vi "CSM - File Loader.vi"(5 "Init State(\"Macro: Initialize\")":string="Macro: Initialize", 7 "Name(\"\" to use uuid)":string="CSM Tiny") -> ()   [LabVIEW 2020]
doc: "Template for building CSM Module without User Interface.\n\n<b>Inputs:</b>\n- <b>Name(\"\" to use uuid)</b>: Module Name\n - If Input is \"\", an uuid will be used for module name. The module is marked as stand-alone mode and will not be included in module list.\n - Fi Input end with '#', the module will worked in worker mode. Modules with the same name will shared the same message queue. Any external message will be processed by one of the modules, depends on who is free.\n - Otherwise, the input string will be used as module name, which should be unique in system. CSM will go to \"Critical Error\" state if duplicated module name is used in system.\n\n<b>Outputs:</b>\n - N/A"
uses:
  <userlib>/_NEVSTOP/Communicable State Machine(CSM)/_Support/Priority Queue/Priority Queue.lvclass/Priority Queue.ctl
  a15cecde-ba48-478f-b3ee-ddca9c6ade3a.vi
  45794baa-ad44-4491-a68b-119a749fa817.vi
  8437d9df-e1d6-4259-972b-d18eb56eaa28.vi
  <userlib>/_NEVSTOP/Communicable State Machine(CSM)/_Support/Process/CSMP-Async Call.vi
  <userlib>/_NEVSTOP/Communicable State Machine(CSM)/_Support/GlobalEvent/GEvt-Generate Status Log.vi
  <userlib>/_NEVSTOP/Communicable State Machine(CSM)/_Support/Process/CSMP-Broadcast.vi
  <userlib>/_NEVSTOP/Communicable State Machine(CSM)/_Support/GlobalEvent/GEvt-Generate Interrupt Log.vi
  <userlib>/_NEVSTOP/Communicable State Machine(CSM)/_Support/GlobalEvent/GEvt-Generate Register Log.vi
  <userlib>/_NEVSTOP/Communicable State Machine(CSM)/_Support/Process/CSMP-Register Status.vi
  <userlib>/_NEVSTOP/Communicable State Machine(CSM)/_Support/GlobalEvent/GEvt-Generate Unregister Log.vi
  <userlib>/_NEVSTOP/Communicable State Machine(CSM)/_Support/Process/CSMP-Unregister Status.vi
  <userlib>/_NEVSTOP/Communicable State Machine(CSM)/_Support/Process/CSMP-Sync Call.vi
  <userlib>/_NEVSTOP/Communicable State Machine(CSM)/_Support/CSMQ/_CSMObj-Unlock.vi
  <userlib>/_NEVSTOP/Communicable State Machine(CSM)/_Support/Process/CSMP-PostPostMsg.vi
  <userlib>/_NEVSTOP/Communicable State Machine(CSM)/_Support/Process/CSMP-PostSendMsg.vi
  <userlib>/_NEVSTOP/Communicable State Machine(CSM)/_Support/CSMQ/_CSMObj-Lock State.vi
  <userlib>/_NEVSTOP/Communicable State Machine(CSM)/_Support/Common/Splite Reason String Part.vi
  <userlib>/_NEVSTOP/Communicable State Machine(CSM)/_Support/Common/Trim Single line Text.vi
  <userlib>/_NEVSTOP/Communicable State Machine(CSM)/_Support/CSMQ/_CSMOFGV Release.vi
  <userlib>/_NEVSTOP/Communicable State Machine(CSM)/_Support/Common/Remove Comments from Line.vi
  <userlib>/_NEVSTOP/Communicable State Machine(CSM)/_Support/Common/Splite Single-line Message.vi
  <userlib>/_NEVSTOP/Communicable State Machine(CSM)/_Support/Common/Parse Next Single-line State.vi
  <userlib>/_NEVSTOP/Communicable State Machine(CSM)/_Support/CSMQ/_CSMOFGV Dequeue.vi
  <userlib>/_NEVSTOP/Communicable State Machine(CSM)/_Support/CSMQ/_CSMObj-Log Error if in a Remote Session.vi
  <userlib>/_NEVSTOP/Communicable State Machine(CSM)/_Support/GlobalEvent/GEvt-Generate State Change Log.vi
  <userlib>/_NEVSTOP/Communicable State Machine(CSM)/_Support/GlobalEvent/GEvt-Generate Remaining States Log.vi
  <userlib>/_NEVSTOP/Communicable State Machine(CSM)/_Support/GlobalEvent/GEvt-Generate Module Destroyed Log.vi
  <userlib>/_NEVSTOP/Communicable State Machine(CSM)/_Support/GlobalEvent/GEvt-Generate Complete Log.vi
  <userlib>/_NEVSTOP/Communicable State Machine(CSM)/_Support/GlobalEvent/GEvt-Generate Module Created Log.vi
  <userlib>/_NEVSTOP/Communicable State Machine(CSM)/_Support/Common/Format Timestamp.vi
  <userlib>/_NEVSTOP/Communicable State Machine(CSM)/AdvanceAPI/CSM - Revert Arguments-Safe String.vi
  <userlib>/_NEVSTOP/Communicable State Machine(CSM)/AdvanceAPI/CSM - Make String Arguments Safe.vi
  <userlib>/_NEVSTOP/Communicable State Machine(CSM)/AdvanceAPI/CSM - Break Down Multiple States String.vi
  <userlib>/_NEVSTOP/Communicable State Machine(CSM)/AdvanceAPI/CSM - Compact Multiple States.vi
  <userlib>/_NEVSTOP/Communicable State Machine(CSM)/_Support/CSMQ/_CSMObj-Message Check.vi
  <userlib>/_NEVSTOP/Communicable State Machine(CSM)/_Support/CSMQ/_CSMObj-Enqueue Cross-Module Message.vi
  <userlib>/_NEVSTOP/Communicable State Machine(CSM)/_Support/CSMQ/_CSMOFGV Get.vi
  <userlib>/_NEVSTOP/Communicable State Machine(CSM)/_Support/FGV-BroadcastRegistry/Cache-Broadcast Registry Search Result.vi
  <userlib>/_NEVSTOP/Communicable State Machine(CSM)/AdvanceAPI/CSM - Register Status Change.vi
  <userlib>/_NEVSTOP/Communicable State Machine(CSM)/AdvanceAPI/CSM - Unregister Status Change.vi
  <userlib>/_NEVSTOP/Communicable State Machine(CSM)/_Support/Common/Hex Str to U8 Data.vi
  <userlib>/_NEVSTOP/Communicable State Machine(CSM)/_Support/Common/Concatenate State with Arguments.vi
  <userlib>/_NEVSTOP/Communicable State Machine(CSM)/_Support/Common/U8 Data to Hex Str.vi
  <userlib>/_NEVSTOP/Communicable State Machine(CSM)/_Support/Priority Queue/Dequeue Element.vi
  <userlib>/_NEVSTOP/Communicable State Machine(CSM)/AdvanceAPI/CSM - Keywords.vi
  <userlib>/_NEVSTOP/Communicable State Machine(CSM)/_Support/Priority Queue/Enqueue Element.vi
  <userlib>/_NEVSTOP/Communicable State Machine(CSM)/_Support/GlobalEvent/FGV-GlobalEventRef.vi
  <userlib>/_NEVSTOP/Communicable State Machine(CSM)/_Support/CSMQ/_CSMOFGV Obtain.vi
  <userlib>/_NEVSTOP/Communicable State Machine(CSM)/_Support/CSMQ/_CSMOFGV.vi
  <userlib>/_NEVSTOP/Communicable State Machine(CSM)/_Support/Error/CSM Not Allowed Message.vi
  <userlib>/_NEVSTOP/Communicable State Machine(CSM)/_Support/GlobalEvent/FGV-StatusChangeEventRef.vi
  <userlib>/_NEVSTOP/Communicable State Machine(CSM)/_Support/FGV-BroadcastRegistry/global-CSMQ FGV Change Flag.vi
  <userlib>/_NEVSTOP/Communicable State Machine(CSM)/_Support/FGV-BroadcastRegistry/global-Broadcast Cache Change Flag.vi
  <userlib>/_NEVSTOP/Communicable State Machine(CSM)/_Support/BroadcastRegistry/HelperVI/Broadcast Item Key.vi
  <userlib>/_NEVSTOP/Communicable State Machine(CSM)/_Support/FGV-BroadcastRegistry/FGV-BroadcastRegistry.vi
  <userlib>/_NEVSTOP/Communicable State Machine(CSM)/_Support/Message/Parse Register Message.vi
  <userlib>/_NEVSTOP/Communicable State Machine(CSM)/_Support/Message/Parse Unregister Message.vi
  <userlib>/_NEVSTOP/Communicable State Machine(CSM)/AdvanceAPI/CSM - Replace Substitution Marks in Messages.vi
  <userlib>/_NEVSTOP/Communicable State Machine(CSM)/addons/API-String-Arugments-Support/_Support/Convert API String Arguments to Data(variant).vi
  <userlib>/_NEVSTOP/Communicable State Machine(CSM)/addons/MassData-Parameter/_support/FGV-MassData.vi
  <userlib>/_NEVSTOP/Communicable State Machine(CSM)/Communicable State Machine.lvlib
  <userlib>/_NEVSTOP/Communicable State Machine(CSM)/addons/Loop-Support/CSM Loop Support.lvlib
panel:
  out "Snippets Count":i32
  out "text":string
  out "offset (in bytes)":i64 format="%.3p"
  out "size (in bytes)":i64 format="%.3p"
  out "State History":string
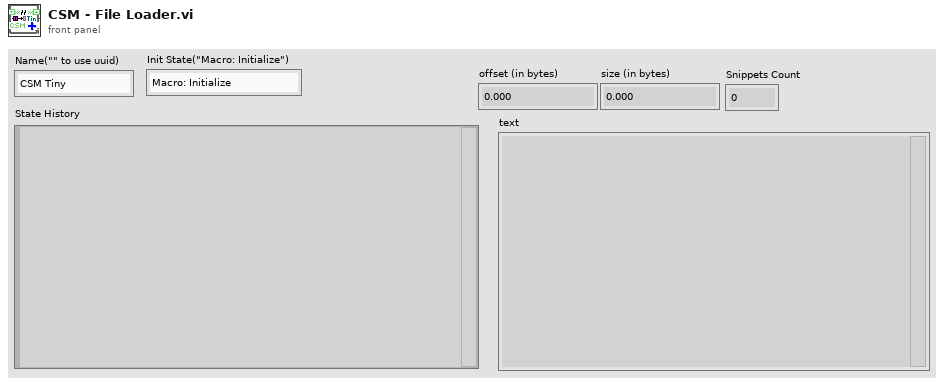
[diagram p1: front panel]
types:
  T1 = enum32{"Invalid", "Standard", "Closed", "Hidden", "Minimized", "Maximized"}
  T2 = enum32{"invalid app kind", "Development System", "Run Time System", "Student Edition", "Embedded LabVIEW", "Evaluation", "Custom"}
  T3 = typedef "Communicable State Machine.lvlib/_CSM_Response Source Message.ctl" = cluster{"‘State":string, "’Arguments":string, "’Error":errorcluster}
  T4 = cluster{"Core":cluster{"Current VI Reference":refnum<vi>, "Close Panel on Exit?":bool}, "Snippets Size":i32, "temp":string, "Snippets Count":i32}
  T5 = cluster{"Current VI Reference":refnum<vi>, "Close Panel on Exit?":bool}
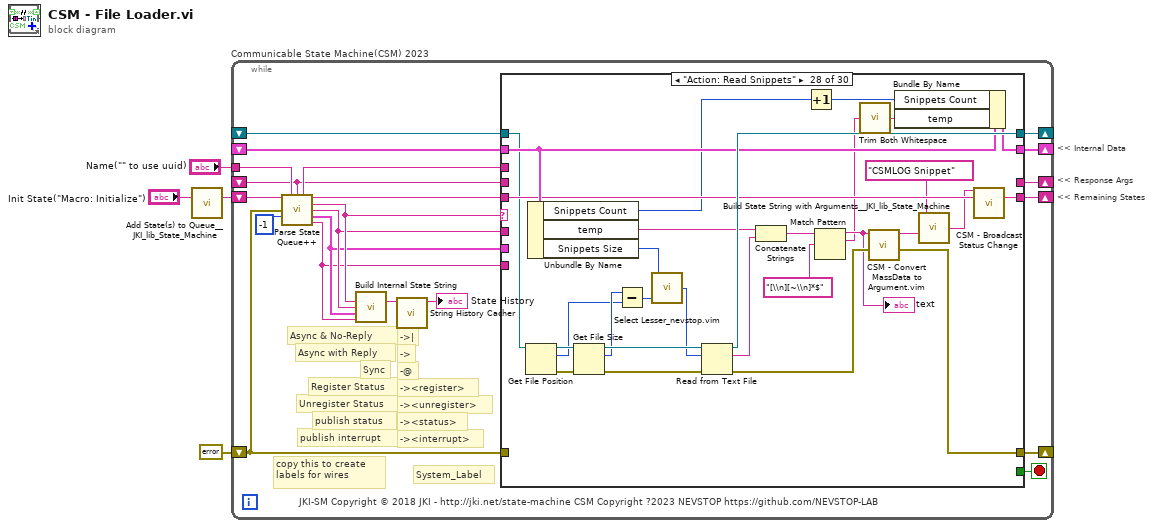
[diagram p0: block diagram]
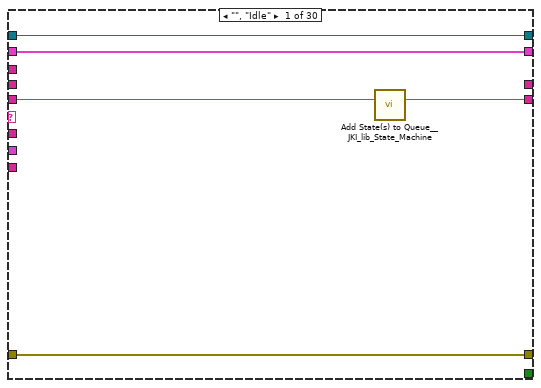
[diagram p2: hidden frame]
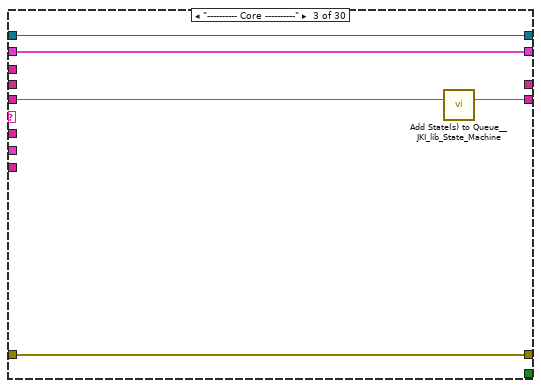
[diagram p4: hidden frame]
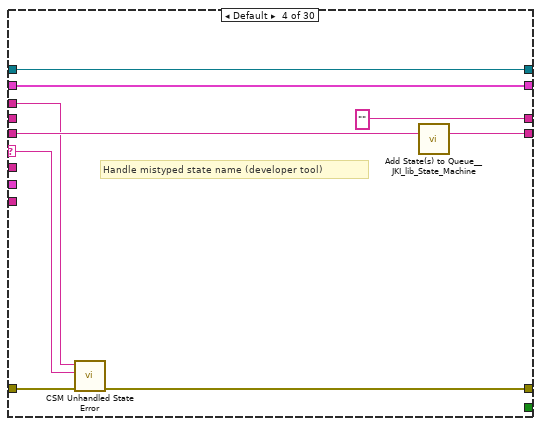
[diagram p5: hidden frame]
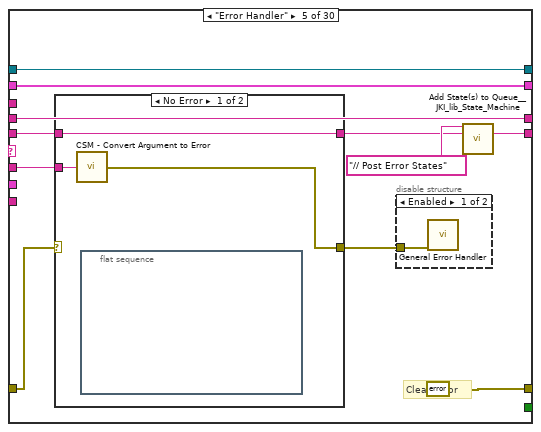
[diagram p6: hidden frame]
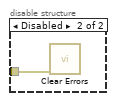
[diagram p7: hidden frame]
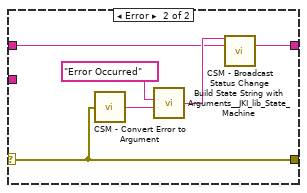
[diagram p8: hidden frame]
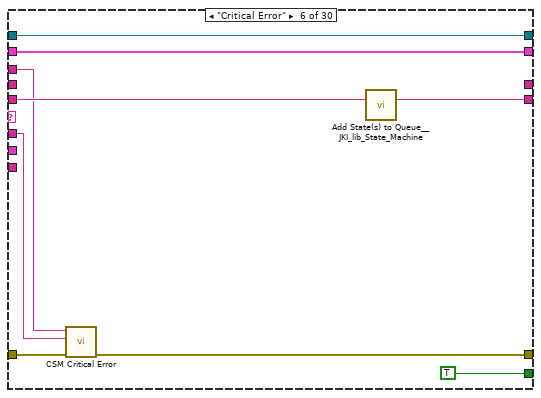
[diagram p9: hidden frame]
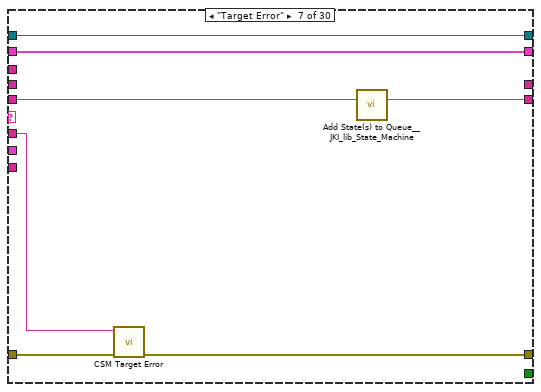
[diagram p10: hidden frame]
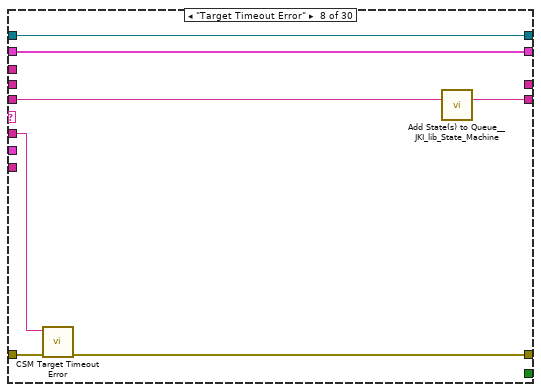
[diagram p11: hidden frame]
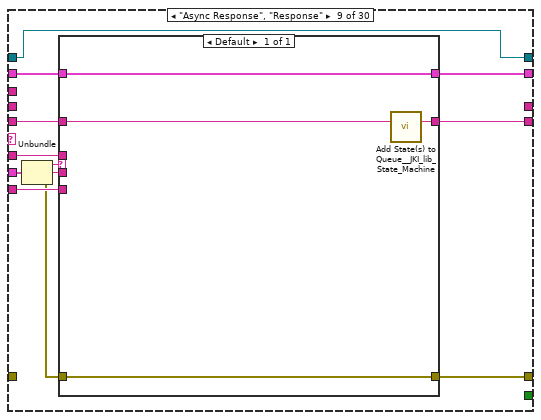
[diagram p12: hidden frame]
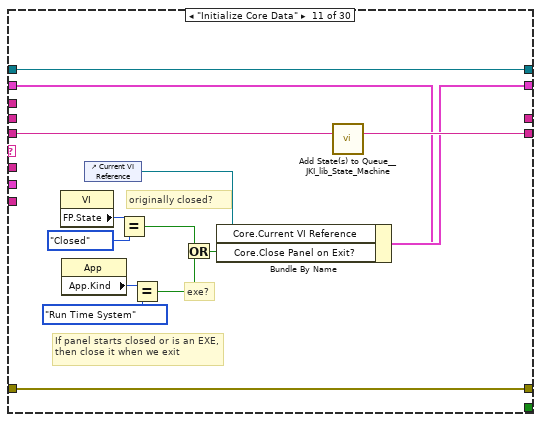
[diagram p14: hidden frame]
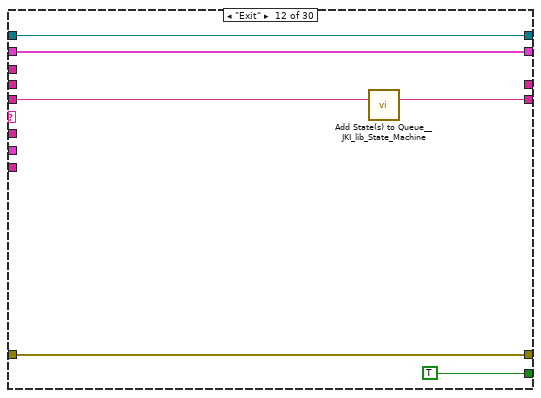
[diagram p15: hidden frame]
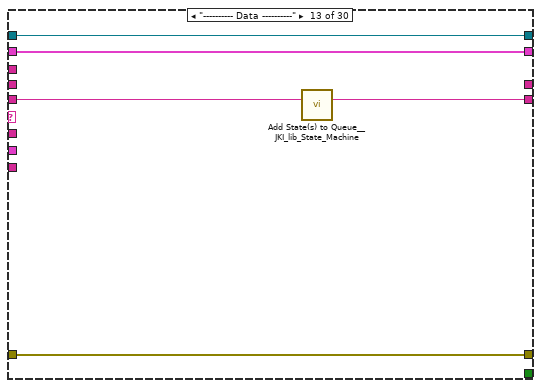
[diagram p16: hidden frame]
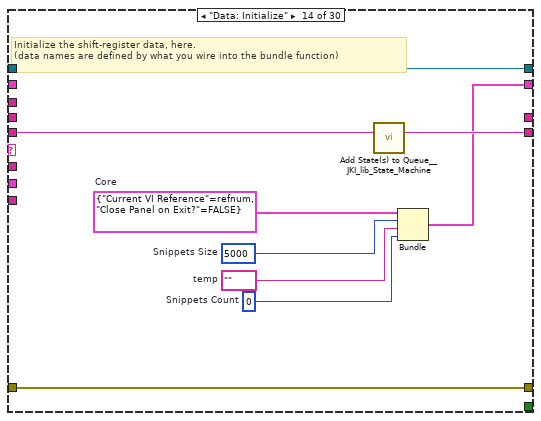
[diagram p17: hidden frame]
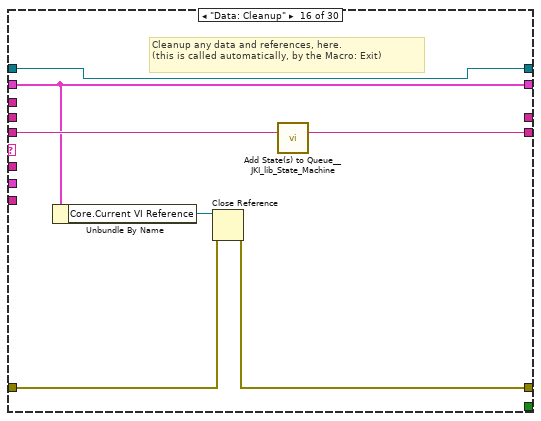
[diagram p19: hidden frame]
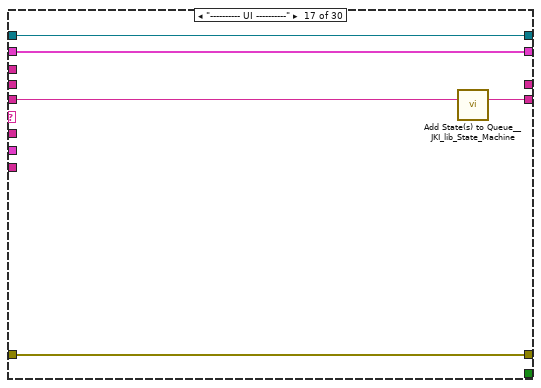
[diagram p20: hidden frame]
diagram:
  # "<< Internal Data"
  # "<< Response Args"
  # "<< Remaining States"
  n1 = call <vilib>:"Add State(s) to Queue__JKI_lib_State_Machine.vi"("State(s) in (\"\")"="Init State(\"Macro: Initialize\")") -> ("States Out"=w4:string)  [unwired: 14 in]
  n2 = while "Communicable State Machine(CSM) 2023" {
    shift-right: [w20] -> _
    shift-left: _ -> [w19]
    shift-right: [w23] -> _
    shift-left: errorcluster {"status"=FALSE, "code"=0, "source"=""} ("error out") -> [w18]
    shift-right: [w22] -> _
    shift-left: w4 -> [w24]
    tunnel: "Name(\"\" to use uuid)" -> [w16]
    shift-right: [w17] -> _
    shift-left: _ -> [w8]
    shift-right: [w6] -> _
    shift-left: _ -> [w5]
    stop <- w21 stop-if-true
    # "-><interrupt>"
    # "-><status>"
    # "-><unregister>"
    # "-><register>"
    # "-@"
    # "->"
    # "->|"
    # "publish interrupt"
    # "publish status"
    # "Unregister Status"
    # "Register Status"
    # "Sync"
    # "Async with Reply"
    # "Async & No-Reply"
    # "copy this to create labels for wires"
    # "System_Label"
    # "JKI-SM Copyright © 2018 JKI - http://jki.net/state-machine CSM Copyright ?2023 NEVSTOP https://github.com/NEVSTOP-LAB"
    n3 = call <userlib>:"Parse State Queue++.vi"("State Queue"=w24, "Name(\"\" to use uuid)"=w16, "Response Arguments"=w8, "Error In (no error)"=w18, "Dequeue Timeout(0ms)"=-1 ("Timeout")) -> ("Name Used"=w9:string, "Remaining States"=w25:string, "Current State"=w13:string, "Arguments"=w12:string, ">> Response Source Message >>"=w11:T3, ">> Source CSM >>"=w10:string)  [unwired: 5 in]
    n4 = call <userlib>:"Build Internal State String.vi"("State"=w13, "Arguments (\"\")"=w12, ">> Response Source Message >>"=w11, "Source (\"\")"=w10) -> ("State with Arguments"=w14:string)  [unwired: 11 in]
    n5 = call <userlib>:"String History Cacher.vi"("String"=w14) -> ("String Cache"=→"State History":string)  [unwired: 10 in]
    n6 = case shown="\"Action: Read Snippets\"" w13 {
      selector: w13 -> [_ _ _ w43 _ _ _ _ _ _ _ _ _ _ _ _ _ _ _ _ _ _ _ _ _ _ _ _ w346 _]
      tunnel: w25 -> [w27 w33 w39 w47 w55 w77 w84 w91 w100 w112 w127 w133 w138 w147 w150 w158 w163 w168 w175 w191 w261 w267 w275 w278 w288 w294 w305 w331 w348 w359]
      tunnel: w12 -> [_ _ _ _ w54 w73 w83 w89 w99 _ _ _ _ _ _ _ _ _ w170 w185 _ _ _ _ w282 _ w295 _ _ _]
      tunnel: w19 -> [w28 w32 w36 w45 w58 w78 w85 w92 w102 w111 w120 w131 w135 _ w149 w153 w160 w166 w173 w187 w258 w264 w272 w277 w287 w291 w303 w333 w336 w357]
      tunnel: [w29 w34 w37 w41 errorcluster {"status"=FALSE, "code"=0, "source"=""} ("error out") w74 w81 w88 w105 w113 w124 w130 w136 w144 w151 w154 w161 w165 w171 w188 w259 w265 w273 w279 w289 w292 w300 w329 w339 w355] -> w23
      tunnel: w18 -> [w29 w34 w37 w48 w56 w79 w82 w90 _ w113 w124 w130 w136 w144 w151 w155 w161 w165 w172 w189 w259 w265 w273 w279 w289 w292 _ _ _ _]
      tunnel: [w30 w33 w38 w46 w51 w76 w86 w93 w101 w112 w126 w132 w137 w146 w150 w157 w162 w167 w174 w190 w260 w266 w274 w278 w285 w293 w304 w332 w347 w358] -> w22
      tunnel: [_ _ _ _ _ TRUE _ _ _ _ _ TRUE _ _ _ _ _ _ _ _ _ _ _ _ _ _ _ _ _ _] -> w21
      tunnel: [w28 w32 w36 w45 w58 w78 w85 w92 w103 w111 w125 w131 w135 w145 w149 w153 w160 w166 w173 w187 w258 w264 w272 w277 w281 w291 w303 w314 w336 w357] -> w20
      tunnel: w10 -> [_ _ _ _ _ _ _ _ w97 _ _ _ _ _ _ _ _ _ _ _ _ _ _ _ _ _ _ _ _ _]
      tunnel: w11 -> [_ _ _ _ _ _ _ _ w104 _ _ _ _ _ _ _ _ _ _ _ _ _ _ _ _ _ _ _ _ _]
      tunnel: [_ _ _ "" w50 _ _ _ _ _ _ _ _ _ _ _ _ _ _ _ _ _ _ _ _ _ _ _ _ _] -> w17
      tunnel: w9 -> [_ _ _ w42 _ w72 _ _ _ _ _ _ _ _ _ _ _ _ _ _ _ _ _ _ _ _ _ _ _ _]
      tunnel: w8 -> [_ _ _ _ w50 _ _ _ _ _ _ _ _ _ _ _ _ _ _ _ _ _ _ _ _ _ _ _ _ _]
      tunnel: [w26 w31 w35 w40 w49 w71 w80 w87 w94 w110 w114 w128 w134 w141 w148 w152 w159 w164 w169 w184 w257 w262 w268 w276 w286 w290 w299 w334 w345 refnum<file> refnum ("refnum out")] -> w6
      tunnel: w5 -> [w26 w31 w35 w40 w49 w71 w80 w87 w94 w110 w114 w128 w134 w141 w148 w152 w159 w164 w169 w184 w257 w262 w268 w276 w286 w290 _ w326 w344 w356]
      frame "", "Idle" {
        n7 = call <vilib>:"Add State(s) to Queue__JKI_lib_State_Machine.vi"("State(s) in (\"\")"=w27) -> ("States Out"=w30:string)  [unwired: 14 in]
      }
      frame "CSM Documentation" {
      }
      frame "---------- Core ----------" {
        n8 = call <vilib>:"Add State(s) to Queue__JKI_lib_State_Machine.vi"("State(s) in (\"\")"=w39) -> ("States Out"=w38:string)  [unwired: 14 in]
      }
      frame Default {
        # "Handle mistyped state name (developer tool)"
        n9 = call <userlib>:"CSM Unhandled State Error.vi"("error in (no error)"=w48, "State"=w43, "CSM"=w42) -> ("error out"=w41:errorcluster)  [unwired: 8 in]
        n10 = call <vilib>:"Add State(s) to Queue__JKI_lib_State_Machine.vi"("State(s) in (\"\")"=w47) -> ("States Out"=w46:string)  [unwired: 14 in]
      }
      frame "Error Handler" {
        # "Clear error"
        n11 = case shown="No Error" w56 {
          selector: w56 -> [_ w65]
          tunnel: [w64 w67] -> w52
          tunnel: w55 -> [w64 w66]
          tunnel: w54 -> [w63 _]
          tunnel: [w62 w65] -> w57
          frame No Error {
            n12 = call <userlib>:"CSM - Convert Argument to Error.vi"("Argument"=w63) -> ("error"=w62:errorcluster)  [unwired: 4 in]
            n13 = flat-sequence {
              frame #0 {
              }
            }
          }
          frame Error {
            n14 = call <userlib>:"CSM - Convert Error to Argument.vi"("error in (no error)"=w65) -> ("Arguments"=w69:string)  [unwired: 4 in]
            n15 = call <vilib>:"Build State String with Arguments__JKI_lib_State_Machine.vi"("Arguments (\"\")"=w69, "State"="Error Occurred" ("Status with Arguments")) -> ("State with Arguments"=w68:string)  [unwired: 4 in]
            n16 = call <userlib>:"CSM - Broadcast Status Change.vi"("Status with Arguments"=w68, "State Queue"=w66) -> ("Remaining States"=w67:string)  [unwired: 13 in]
          }
        }
        n17 = disable-structure shown="Enabled" {
          disable-tunnel: w57 -> [w60 w61]
          frame Enabled {
            n18 = call <vilib>:"General Error Handler.vi"("error in (no error)"=w60) -> ()  [unwired: 10 in, 5 out]
          }
          frame Disabled {
            n19 = call <vilib>:"Clear Errors.vi"("error in (no error)"=w61) -> ()  [unwired: 5 in, 2 out]
          }
        }
        n20 = call <vilib>:"Add State(s) to Queue__JKI_lib_State_Machine.vi"("State(s) in Front (\"\")"="// Post Error States", "State(s) in (\"\")"=w52) -> ("States Out"=w51:string)  [unwired: 13 in]
      }
      frame "Critical Error" {
        n21 = call <userlib>:"CSM Critical Error.vi"("error in (no error)"=w79, "input"=w73, "CSM Name"=w72) -> ("error out"=w74:errorcluster)  [unwired: 8 in]
        n22 = call <vilib>:"Add State(s) to Queue__JKI_lib_State_Machine.vi"("State(s) in (\"\")"=w77) -> ("States Out"=w76:string)  [unwired: 14 in]
      }
      frame "Target Error" {
        n23 = call <userlib>:"CSM Target Error.vi"("error in (no error)"=w82, "CSM Name"=w83) -> ("error out"=w81:errorcluster)  [unwired: 9 in]
        n24 = call <vilib>:"Add State(s) to Queue__JKI_lib_State_Machine.vi"("State(s) in (\"\")"=w84) -> ("States Out"=w86:string)  [unwired: 14 in]
      }
      frame "Target Timeout Error" {
        n25 = call <userlib>:"CSM Target Timeout Error.vi"("error in (no error)"=w90, "CSM Name"=w89) -> ("error out"=w88:errorcluster)  [unwired: 9 in]
        n26 = call <vilib>:"Add State(s) to Queue__JKI_lib_State_Machine.vi"("State(s) in (\"\")"=w91) -> ("States Out"=w93:string)  [unwired: 14 in]
      }
      frame "Async Response", "Response" {
        n27 = Unbundle(w104) -> ("‘State"=w98:string, "’Arguments"=w96:string, "’Error"=w95:errorcluster)
        n28 = case shown="Default" w98 {
          tunnel: [w109] -> w105
          tunnel: w95 -> [w109]
          tunnel: [w108] -> w103
          tunnel: w102 -> [w108]
          tunnel: [w106] -> w101
          tunnel: w100 -> [w107]
          tunnel: w99 -> [_]
          tunnel: w97 -> [_]
          tunnel: w96 -> [_]
          frame Default {
            n29 = call <vilib>:"Add State(s) to Queue__JKI_lib_State_Machine.vi"("State(s) in (\"\")"=w107) -> ("States Out"=w106:string)  [unwired: 14 in]
          }
        }
      }
      frame "Async Message Posted" {
      }
      frame "Initialize Core Data" {
        # "originally closed?"
        # "exe?"
        # "If panel starts closed or is an EXE, then close it when we exit"
        n30 = property class="VI"() -> ("FP.State"=w117:T1)  [unwired: 2 in, 2 out]
        n31 = property class="App"() -> ("App.Kind"=w123:T2)  [unwired: 2 in, 2 out]
        n32 = control-ref of="Current VI Reference"() -> (w118:refnum<vi>)
        n33 = Equal?(x=w117, y=T1."Closed" ("Front Panel Window:State")) -> (x = y?=w115:bool)
        n34 = Equal?(x=w123, y=T2."Run Time System" ("Application:Kind")) -> (x = y?=w121:bool)
        n35 = Or(x=w115, y=w121) -> (x .or. y?=w119:bool)
        n36 = Bundle By Name(cluster=w120, "Core.Current VI Reference"=w118, "Core.Close Panel on Exit?"=w119) -> (w125:T4)
        n37 = call <vilib>:"Add State(s) to Queue__JKI_lib_State_Machine.vi"("State(s) in (\"\")"=w127) -> ("States Out"=w126:string)  [unwired: 14 in]
      }
      frame "Exit" {
        n38 = call <vilib>:"Add State(s) to Queue__JKI_lib_State_Machine.vi"("State(s) in (\"\")"=w133) -> ("States Out"=w132:string)  [unwired: 14 in]
      }
      frame "---------- Data ----------" {
        n39 = call <vilib>:"Add State(s) to Queue__JKI_lib_State_Machine.vi"("State(s) in (\"\")"=w138) -> ("States Out"=w137:string)  [unwired: 14 in]
      }
      frame "Data: Initialize" {
        w139 = 0  # Snippets Count
        w140 = ""  # temp
        w142 = T5 {"Current VI Reference"=refnum, "Close Panel on Exit?"=FALSE}  # Core
        w143 = 5000  # Snippets Size
        # "Initialize the shift-register data, here.\n(data names are defined by what you wire into the bundle function)"
        n40 = call <vilib>:"Add State(s) to Queue__JKI_lib_State_Machine.vi"("State(s) in (\"\")"=w147) -> ("States Out"=w146:string)  [unwired: 14 in]
        n41 = Bundle("Core"=w142, "Snippets Size"=w143, "temp"=w140, "Snippets Count"=w139) -> (w145:T4)  [unwired: 1 in]
      }
      frame "Data: Update Indicators" {
      }
      frame "Data: Cleanup" {
        # "Cleanup any data and references, here.\n(this is called automatically, by the Macro: Exit)"
        n42 = Unbundle By Name(w153) -> ("Core.Current VI Reference"=w156:refnum<vi>)
        n43 = Close Reference(reference=w156, error in (no error)=w155) -> (error out=w154:errorcluster)
        n44 = call <vilib>:"Add State(s) to Queue__JKI_lib_State_Machine.vi"("State(s) in (\"\")"=w158) -> ("States Out"=w157:string)  [unwired: 14 in]
      }
      frame "---------- UI ----------" {
        n45 = call <vilib>:"Add State(s) to Queue__JKI_lib_State_Machine.vi"("State(s) in (\"\")"=w163) -> ("States Out"=w162:string)  [unwired: 14 in]
      }
      frame "UI: Initialize" {
        n46 = call <vilib>:"Add State(s) to Queue__JKI_lib_State_Machine.vi"("State(s) in (\"\")"=w168) -> ("States Out"=w167:string)  [unwired: 14 in]
      }
      frame "UI: Cursor Set" {
        # "Argument"
        n47 = disable-structure shown="TARGET_TYPE!=Windows" {
          disable-tunnel: w172 -> [w178 w183]
          disable-tunnel: [w177 w183] -> w171
          disable-tunnel: w170 -> [w176 _]
          frame condition #0 (active) {
            n48 = case shown="\"Idle\", Default" w176 {
              tunnel: w178 -> [w180 w182]
              tunnel: [w179 w181] -> w177
              frame "Idle", Default {
                n49 = call <vilib>:"Unset Busy.vi"("error in (no error)"=w180) -> ("error out"=w179:errorcluster)  [unwired: 10 in]
              }
              frame "Busy" {
                n50 = call <vilib>:"Set Busy.vi"("error in (no error)"=w182) -> ("error out"=w181:errorcluster)  [unwired: 9 in, 1 out]
              }
            }
          }
          frame condition #1 {
          }
        }
        n51 = call <vilib>:"Add State(s) to Queue__JKI_lib_State_Machine.vi"("State(s) in (\"\")"=w175) -> ("States Out"=w174:string)  [unwired: 14 in]
      }
      frame "UI: Front Panel State" {
        # "Argument"
        n52 = Unbundle By Name(w187) -> ("Core.Current VI Reference"=w186:refnum<vi>)
        n53 = call <vilib>:"Add State(s) to Queue__JKI_lib_State_Machine.vi"("State(s) in (\"\")"=w191) -> ("States Out"=w190:string)  [unwired: 14 in]
        n54 = case shown="\"Close\", \"Closed\"" w185 {
          tunnel: w189 -> [w197 w212 w223 w236 w249]
          tunnel: [w199 w213 w225 w238 w251] -> w188
          tunnel: w186 -> [w198 w210 w224 w237 w250]
          frame "Open", "Standard", Default {
            w192 = T1."Standard" ("State")
            n55 = property class="VI"(reference=w198, error in=w197) -> (reference out=w195:refnum<vi>, error out=w196:errorcluster, "FP.State"=w194:T1)
            n56 = Not Equal?(x=w194, y=w192) -> (x != y?=w193:bool)
            n57 = case shown="True" w193 {
              tunnel: [w203 w205] -> w199
              tunnel: w196 -> [w202 w205]
              tunnel: w195 -> [w201 _]
              tunnel: w192 -> [w200 _]
              frame True {
                n58 = invoke class="VI" method="FP.Open"(reference=w201, error in=w202, "Activate"=TRUE, "State"=w200) -> (error out=w203:errorcluster)  [unwired: 1 in, 4 out]
              }
              frame False {
              }
            }
          }
          frame "Close", "Closed" {
            n59 = property class="VI"(reference=w210, error in=w212) -> (reference out=w209:refnum<vi>, error out=w211:errorcluster, "FP.State"=w207:T1)
            n60 = Not Equal?(x=w207, y=T1."Closed" ("Front Panel Window:State")) -> (x != y?=w206:bool)
            n61 = case shown="False" w206 {
              tunnel: [w214 w217] -> w213
              tunnel: w211 -> [w214 w216]
              tunnel: w209 -> [_ w215]
              frame False {
              }
              frame True {
                n62 = invoke class="VI" method="FP.Close"(reference=w215, error in=w216) -> (error out=w217:errorcluster)  [unwired: 1 in, 2 out]
              }
            }
          }
          frame "Hidden", "Hide" {
            w218 = T1."Hidden" ("State")
            n63 = property class="VI"(reference=w224, error in=w223) -> (reference out=w221:refnum<vi>, error out=w222:errorcluster, "FP.State"=w220:T1)
            n64 = Not Equal?(x=w220, y=w218) -> (x != y?=w219:bool)
            n65 = case shown="True" w219 {
              tunnel: [w229 w230] -> w225
              tunnel: w222 -> [w228 w230]
              tunnel: w221 -> [w227 _]
              tunnel: w218 -> [w226 _]
              frame True {
                n66 = invoke class="VI" method="FP.Open"(reference=w227, error in=w228, "State"=w226) -> (error out=w229:errorcluster)  [unwired: 2 in, 4 out]
              }
              frame False {
              }
            }
          }
          frame "Minimize", "Minimized" {
            w231 = T1."Minimized" ("State")
            n67 = property class="VI"(reference=w237, error in=w236) -> (reference out=w234:refnum<vi>, error out=w235:errorcluster, "FP.State"=w233:T1)
            n68 = Not Equal?(x=w233, y=w231) -> (x != y?=w232:bool)
            n69 = case shown="True" w232 {
              tunnel: [w242 w243] -> w238
              tunnel: w235 -> [w241 w243]
              tunnel: w234 -> [w240 _]
              tunnel: w231 -> [w239 _]
              frame True {
                n70 = invoke class="VI" method="FP.Open"(reference=w240, error in=w241, "State"=w239) -> (error out=w242:errorcluster)  [unwired: 2 in, 4 out]
              }
              frame False {
              }
            }
          }
          frame "Maximize", "Maximized" {
            w244 = T1."Maximized" ("State")
            n71 = property class="VI"(reference=w250, error in=w249) -> (reference out=w247:refnum<vi>, error out=w248:errorcluster, "FP.State"=w246:T1)
            n72 = Not Equal?(x=w246, y=w244) -> (x != y?=w245:bool)
            n73 = case shown="True" w245 {
              tunnel: [w255 w256] -> w251
              tunnel: w248 -> [w254 w256]
              tunnel: w247 -> [w253 _]
              tunnel: w244 -> [w252 _]
              frame True {
                n74 = invoke class="VI" method="FP.Open"(reference=w253, error in=w254, "State"=w252) -> (error out=w255:errorcluster)  [unwired: 2 in, 4 out]
              }
              frame False {
              }
            }
          }
        }
      }
      frame "---------- Macro ----------" {
        n75 = call <vilib>:"Add State(s) to Queue__JKI_lib_State_Machine.vi"("State(s) in (\"\")"=w261) -> ("States Out"=w260:string)  [unwired: 14 in]
      }
      frame "Macro: Initialize" {
        n76 = call <vilib>:"Add State(s) to Queue__JKI_lib_State_Machine.vi"("State(s) in Front (\"\")"="Data: Initialize\nInitialize Core Data\nData: Update Indicators", "State(s) in (\"\")"=w267) -> ("States Out"=w266:string)  [unwired: 13 in]
      }
      frame "Macro: Exit" {
        n77 = call <vilib>:"Add State(s) to Queue__JKI_lib_State_Machine.vi"("State(s) in Front (\"\")"="//Exit Sub-Modules ", "State(s) at Back (\"\")"="Data: Cleanup\nExit") -> ("States Out"=w270:string)  [unwired: 13 in]
        n78 = call <vilib>:"Add State(s) to Queue__JKI_lib_State_Machine.vi"("State(s) in Front (\"\")"=w270, "State(s) in (\"\")"=w275) -> ("States Out"=w274:string)  [unwired: 13 in]
      }
      frame "---------- API ----------" {
      }
      frame "API: Load CSMLOG File" {
        n79 = Bundle By Name(cluster=w287, "Snippets Count"=0) -> (w281:T4)
        n80 = call-poly <userlib>:"Build Message with Arguments++.vi"("States with Replace Token"="Action: Open File >> <param>\nAction: Continue Check -><loop>\nAction: Close File\nMacro: Exit " ("States Out in"), "<param>"=w282) -> ("States"=w284:string)  [unwired: 13 in]
        n81 = call <userlib>:"CSMLS - Define Loop State(s).vi"("States Out in"=w284, "Remaining States"=w288) -> ("States Out out"=w285:string)  [unwired: 13 in]
      }
      frame "---------- Action ----------" {
        n82 = call <vilib>:"Add State(s) to Queue__JKI_lib_State_Machine.vi"("State(s) in (\"\")"=w294) -> ("States Out"=w293:string)  [unwired: 14 in]
      }
      frame "Action: Open File" {
        n83 = call "Convert API String Arguments to Data.vim"("Type"=path "" ("file path (use dialog)"), "String"=w295) -> ("error"=w298:errorcluster, "Data"=w296:path)  [unwired: 6 in]
        n84 = Open/Create/Replace File(file path (use dialog)=w296, error in=w298) -> (refnum out=w302:refnum<file>, error out=w301:errorcluster)  [unwired: 4 in, 1 out]
        n85 = Get File Size(file=w302, error in=w301) -> (refnum out=w299:refnum<file>, 0:w300:errorcluster)  [unwired: 1 out]
        n86 = call <vilib>:"Add State(s) to Queue__JKI_lib_State_Machine.vi"("State(s) in (\"\")"=w305) -> ("States Out"=w304:string)  [unwired: 14 in]
      }
      frame "Action: Read Snippets" {
        n87 = Get File Position(7:w326) -> (0:w327:errorcluster, 2:w322:i64, 3:w328:refnum<file>)  [unwired: 1 in]
        n88 = Unbundle By Name(w333) -> ("Snippets Count"=w310:i32, "temp"=w317:string, "Snippets Size"=w320:i32)
        n89 = Get File Size(file=w328, error in=w327) -> (refnum out=w324:refnum<file>, size (in bytes)=w323:i64, 0:w325:errorcluster)
        n90 = Subtract(x=w323, y=w322) -> (x-y=w321:i64)
        n91 = call "Select Lesser_nevstop.vim"("A"=w320, "B"=w321) -> ("lesser"=w319:i64)  [unwired: 3 in]
        n92 = Read from Text File(file (use dialog)=w324, count=w319, error in=w325) -> (refnum out=w334:refnum<file>, text=w318:string, error out=w330:errorcluster)  [unwired: 1 in, 1 out]
        n93 = Concatenate Strings(w317, w318) -> (w316:string)
        n94 = Increment(x=w310) -> (x+1=w309:i32)
        n95 = Match Pattern(string=w316, regular expression="[\\n][~\\n]*$") -> (before substring=w313:string, match substring=w312:string)  [unwired: 1 in, 2 out]
        "text" <- w313
        n96 = call <userlib>:"Trim Both Whitespace.vi"("string"=w312) -> ("trimmed string"=w311:string)  [unwired: 1 in]
        n97 = call "CSM - Convert MassData to Argument.vim"("error in (no error)"=w330, "DBL"=w313) -> ("error out"=w329:errorcluster, "MassData Argument"=w308:string)  [unwired: 6 in]
        n98 = Bundle By Name(cluster=w333, "Snippets Count"=w309, "temp"=w311) -> (w314:T4)
        n99 = call <vilib>:"Build State String with Arguments__JKI_lib_State_Machine.vi"("Arguments (\"\")"=w308, "State"="CSMLOG Snippet") -> ("State with Arguments"=w307:string)  [unwired: 4 in]
        n100 = call <userlib>:"CSM - Broadcast Status Change.vi"("Status with Arguments"=w307, "State Queue"=w331) -> ("Remaining States"=w332:string)  [unwired: 13 in]
      }
      frame "Action: Continue Check" {
        n101 = Get File Position(7:w344) -> (0:w342:errorcluster, 2:w341:i64, 3:w343:refnum<file>)  [unwired: 1 in]
        "offset (in bytes)" <- w341
        n102 = Unbundle By Name(w336) -> ("Snippets Count"=→"Snippets Count":i32)
        n103 = Wait (ms)(milliseconds to wait=u32 1) -> ()  [unwired: 1 out]
        n104 = Get File Size(file=w343, error in=w342) -> (refnum out=w345:refnum<file>, size (in bytes)=w340:i64, 0:w339:errorcluster)
        "size (in bytes)" <- w340
        n105 = Greater Or Equal?(x=w341, y=w340) -> (x >= y?=w338:bool)
        n106 = case shown="False" w338 {
          tunnel: w348 -> [w352 w353]
          tunnel: [w351 w353] -> w347
          tunnel: w346 -> [w350 _]
          frame False {
            n107 = call <userlib>:"CSMLS - Append Continuous State.vi"("Loop State(s) and Arguments"="Action: Read Snippets", "Continous State"=w350, "Remaining States"=w352) -> ("States Out"=w351:string)  [unwired: 8 in]
          }
          frame True {
          }
        }
      }
      frame "Action: Close File" {
        n108 = Close File(refnum=w356) -> (error out=w355:errorcluster)  [unwired: 1 in, 1 out]
        n109 = call <vilib>:"Add State(s) to Queue__JKI_lib_State_Machine.vi"("State(s) in (\"\")"=w359) -> ("States Out"=w358:string)  [unwired: 14 in]
      }
    }
  }
